vi "test_4 (SubVI).vi"(8 "Filename":path=path "C:/Users/Dyakov_AVi/Nextcloud/bioreactor_labview/test_1.lvm", 9 "Numeric":i32, 10 "y":i32=100, 11 "Voltage":dbl) -> ()   [LabVIEW 2016]
uses:
  <vilib>/express/express shared/transition.llb/Dynamic To Waveform Array.vi
  <vilib>/express/express signal manip/GetorSetDDTAttributes/Set DDT Attributes/SetT0.vi
  <vilib>/express/express shared/transition.llb/Waveform Array To Dynamic.vi
  <vilib>/express/express signal manip/GetorSetDDTAttributes/Set DDT Attributes/Set DDT Properties.xnode
  <vilib>/ptbypt/NI_PtbyPt.lvlib
panel:
  out "relative seconds":dbl format="%_19f"
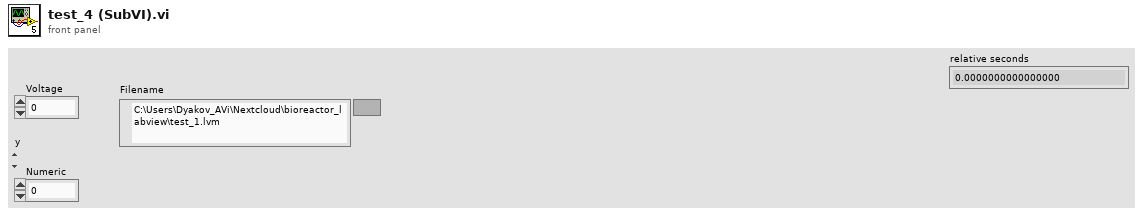
[diagram p1: front panel]
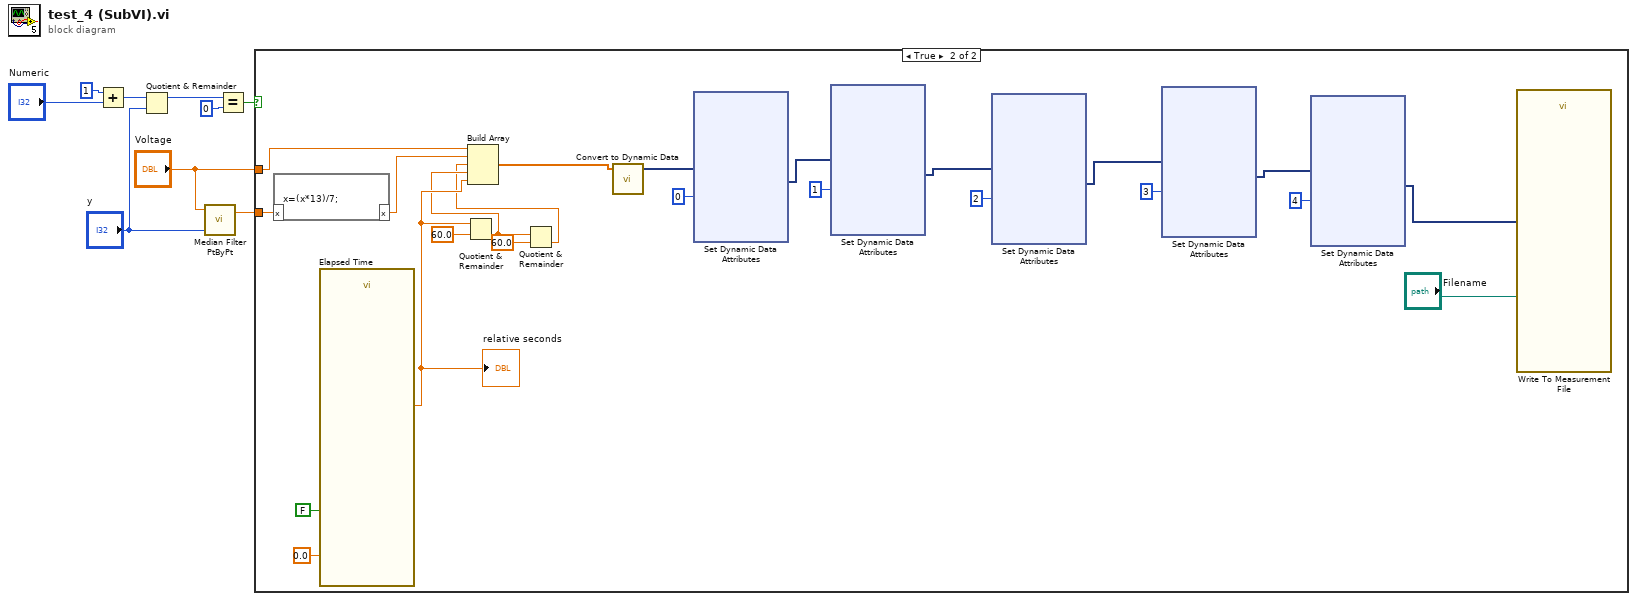
[diagram p0: block diagram]
diagram:
  n1 = Add(x=1, y="Numeric") -> (x+y=w4:i32)
  n2 = Quotient & Remainder(x=w4, y="y") -> (x-y*floor(x/y)=w1:i32)  [unwired: 1 out]
  n3 = call <vilib>:"Median Filter PtByPt.vi"("rank"="y", "x"="Voltage") -> ("Filtered x"=w6:dbl)  [unwired: 2 in, 1 out]
  n4 = Equal?(x=w1, y=0) -> (x = y?=w8:bool)
  n5 = case shown="True" w8 {
    tunnel: w6 -> [_ w32]
    tunnel: "Voltage" -> [_ w30]
    frame False {
    }
    frame True {
      n6 = formula code="x=(x*13)/7;"("x"=w32) -> ("x"=w15:dbl)
      n7 = call "Elapsed Time"("Auto Reset"=FALSE, "Set Start Time (s)"=0.0) -> ("Elapsed Time (s)"=w13:dbl)  [unwired: 10 in, 7 out]
      "relative seconds" <- w13
      n8 = Quotient & Remainder(x=w13, y=60.0) -> (floor(x/y)=w12:dbl)  [unwired: 1 out]
      n9 = Quotient & Remainder(x=w12, y=60.0) -> (floor(x/y)=w10:dbl)  [unwired: 1 out]
      n10 = Build Array(w30, w15, w10, w12, w13) -> (w29:dbl[])
      n11 = call "Convert to Dynamic Data"("Array"=w29) -> ("Dynamic Data Type"=w16:dynamicdata)  [unwired: 3 in]
      n12 = xnode "Set Dynamic Data Attributes"("Signals In"=w16, "Signal Index"=0) -> ("Signals Out"=w28:dynamicdata)  [unwired: 1 in, 1 out]
      n13 = xnode "Set Dynamic Data Attributes"("Signals In"=w28, "Signal Index"=1) -> ("Signals Out"=w23:dynamicdata)  [unwired: 1 in, 1 out]
      n14 = xnode "Set Dynamic Data Attributes"("Signals In"=w23, "Signal Index"=2) -> ("Signals Out"=w22:dynamicdata)  [unwired: 1 in, 1 out]
      n15 = xnode "Set Dynamic Data Attributes"("Signals In"=w22, "Signal Index"=3) -> ("Signals Out"=w21:dynamicdata)  [unwired: 1 in, 1 out]
      n16 = xnode "Set Dynamic Data Attributes"("Signals In"=w21, "Signal Index"=4) -> ("Signals Out"=w20:dynamicdata)  [unwired: 1 in, 1 out]
      n17 = call "Write To Measurement File"("Signals"=w20, "Filename"="Filename") -> ()  [unwired: 15 in, 3 out]
    }
  }
